vi "Adaptive learning.vi"(1 "LRmax":sgl format="%.2f", 2 "RMS (i)":sgl format="%.2f", 3 "LRmin":sgl format="%.2f", 4 "Learn rate":sgl format="%.2f", 5 "Adaptive learning?":bool, 6 "RMS (i-1)":sgl format="%.2f") -> (0 "Learn rate":sgl format="%.2f")   [LabVIEW 2010]
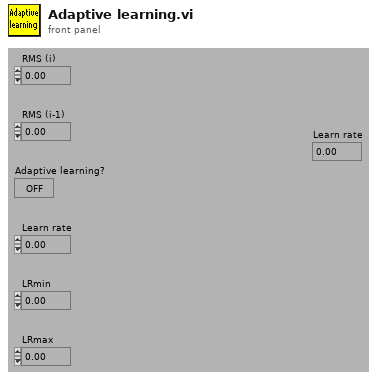
[diagram p1: front panel]
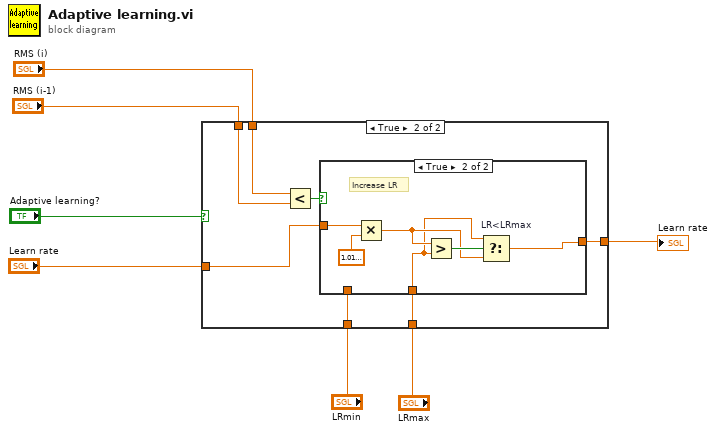
[diagram p0: block diagram]
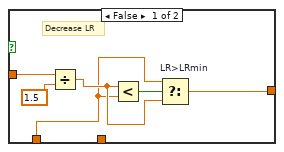
[diagram p3: hidden frame]
diagram:
  n1 = case shown="True" "Adaptive learning?" {
    tunnel: [w8 w14] -> w2
    tunnel: "Learn rate" -> [w8 w13]
    tunnel: "LRmax" -> [_ w12]
    tunnel: "LRmin" -> [_ w11]
    tunnel: "RMS (i)" -> [_ w10]
    tunnel: "RMS (i-1)" -> [_ w9]
    frame False {
    }
    frame True {
      n2 = Less?(x=w10, y=w9) -> (x < y?=w15:bool)
      n3 = case shown="True" w15 {
        tunnel: [w18 w24] -> w14
        tunnel: w13 -> [w17 w23]
        tunnel: w12 -> [_ w22]
        tunnel: w11 -> [w16 _]
        frame False {
          # "Decrease LR"
          n4 = Divide(x=w17, y=sgl 1.5) -> (x/y=w19:sgl)
          n5 = Less?(x=w19, y=w16) -> (x < y?=w20:bool)
          n6 = Select "LR>LRmin"(t=w16, s=w20, f=w19) -> (s? t:f=w18:sgl)
        }
        frame True {
          # "Increase LR"
          n7 = Multiply(x=w23, y=sgl 1.02) -> (x*y=w25:sgl)
          n8 = Greater?(x=w25, y=w22) -> (0:w26:bool)
          n9 = Select "LR<LRmax"(t=w22, s=w26, f=w25) -> (s? t:f=w24:sgl)
        }
      }
    }
  }
  "Learn rate" <- w2
